vi "Configure Ramp Symmetry.vi"(8 "error in (no error)":errorcluster, 10 "Symmetry (100 %)":i32=100 min=0 max=100, 11 "VISA resource name":refnum<visa-resource-name>) -> (0 "error out":errorcluster, 3 "VISA resource name out":refnum<visa-resource-name>)   [LabVIEW 2017, in "Keithley 3390.lvlib"]
doc: "Sets the symmetry of the ramp waveform."
uses:
  Keithley 3390.lvlib
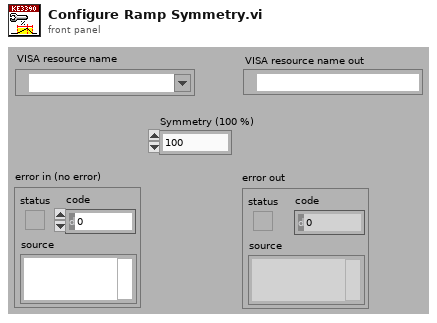
[diagram p1: front panel]
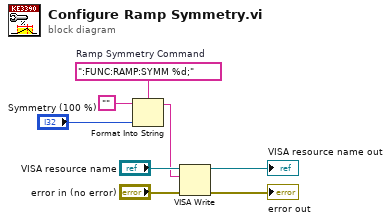
[diagram p0: block diagram]
diagram:
  w4 = ":FUNC:RAMP:SYMM %d;"  # Ramp Symmetry Command
  n1 = Format Into String(format string=w4, initial string="", "Symmetry (100 %)") -> (resulting string=w6:string)  [unwired: 1 in, 1 out]
  n2 = VISA Write(VISA resource name="VISA resource name", write buffer=w6, error in (no error)="error in (no error)") -> (VISA resource name out=→"VISA resource name out":refnum<visa-resource-name>, error out=→"error out":errorcluster)  [unwired: 1 out]
